vi "SerialNo.vi"(0 "DB serial number IN":string, 2 "Run uninterrupted?":bool) -> (6 "DB serial number OUT":string, 7 "Continue?":bool)   [LabVIEW 2018]
uses:
  globals/QC_RunInformation.vi
panel:
  in  "Comments:":string
  in  "DB Serial No.:":string
  in  "Batch No.:":string
  in  "Device Category:":string(combo)="ATLAS18SS"
  in  "Manufacturer:":string(combo)="Hamamatsu"
  in  "Wafer No.:":string
  in  "Cancel":bool
  in  "OK":bool
  # "ATLAS Serial No."
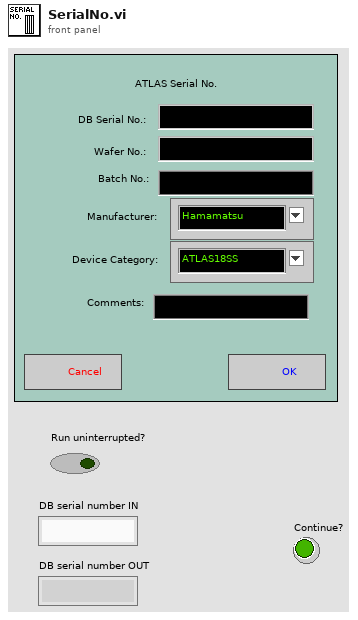
[diagram p1: front panel]
types:
  T1 = cluster{string, string, string, string, string, string, string}
  T2 = cluster{"Institute":string, "Manufacturers":string[], "Devices":string[], "Serialnumbers Lookup DB":string, "Data directory":string, "Backup & screenshot directory":string, "List of known users":string[], "Measurement switch not used":bool, "Measurement Switch":string, "DUT Switch":string, "Rseries IV [MOhm]":string, "Rshunt IV [MOhm]":string, "Rseries CV [MOhm]":string, "DC blocking Cap [µF]":string, "Rseries LCR [MOhm]":string, "Rseries stability [MOhm]":string, "Rshunt stability [MOhm]":string, "Rseries striptest bias [MOhm]":string, "Rseries strip pinhole [MOhm]":string}
  T3 = cluster{"Sensor Serial No.:":string, "Wafer:":string, "Batch:":string, "Manufacturer:":string, "Device Category:":string, "Database Serial No.:":string, "Date Initiated:":string, "Time Initiated:":string, "Test":string, "Probeplan used:":string, "End of Run Status":dbl, "End of Run comment:":string, "User:":string, "Vbias SMU":string, "LCR":string, "Test SMU":string, "Test DMM":string, "Comments":string, "Measurement results":cluster{"IV":string, "CV":string, "Cis":string, "Ris":string, "Stability":string, "PTP":string, "Striptest":string}}
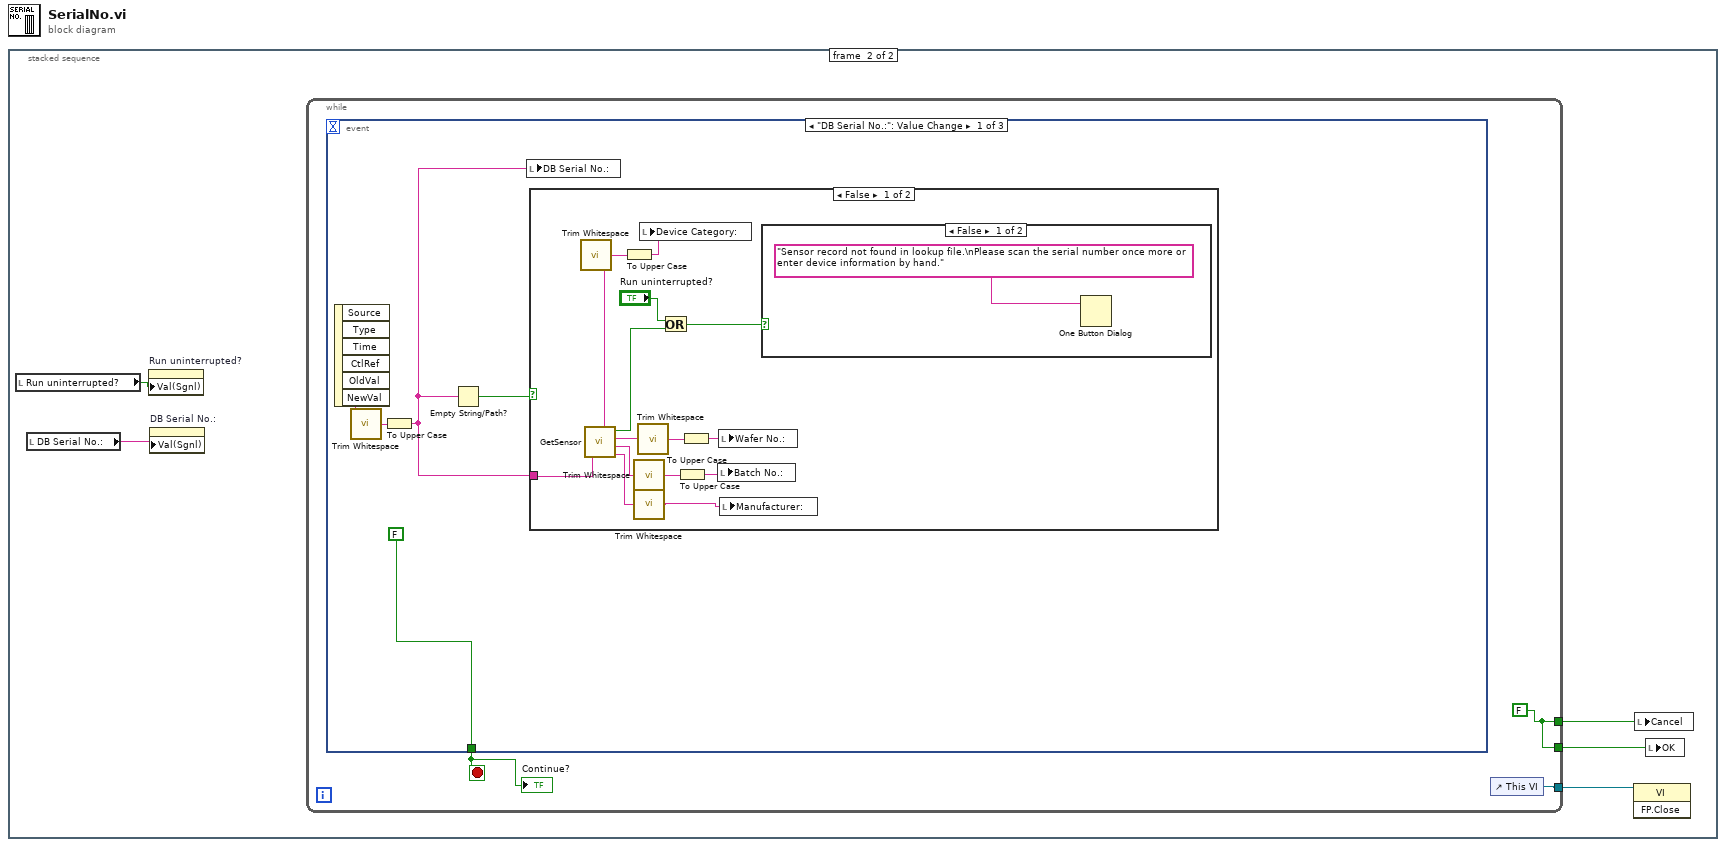
[diagram p0: block diagram]
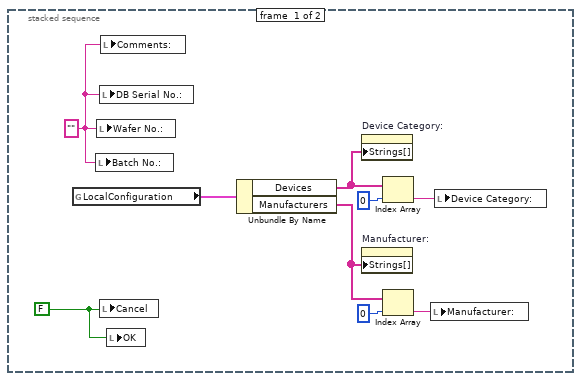
[diagram p2: hidden frame]
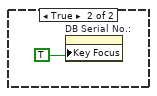
[diagram p4: hidden frame]
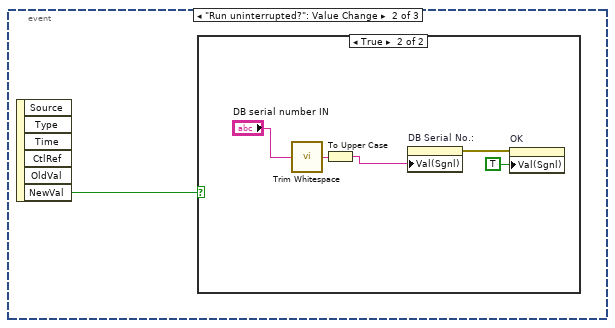
[diagram p5: hidden frame]
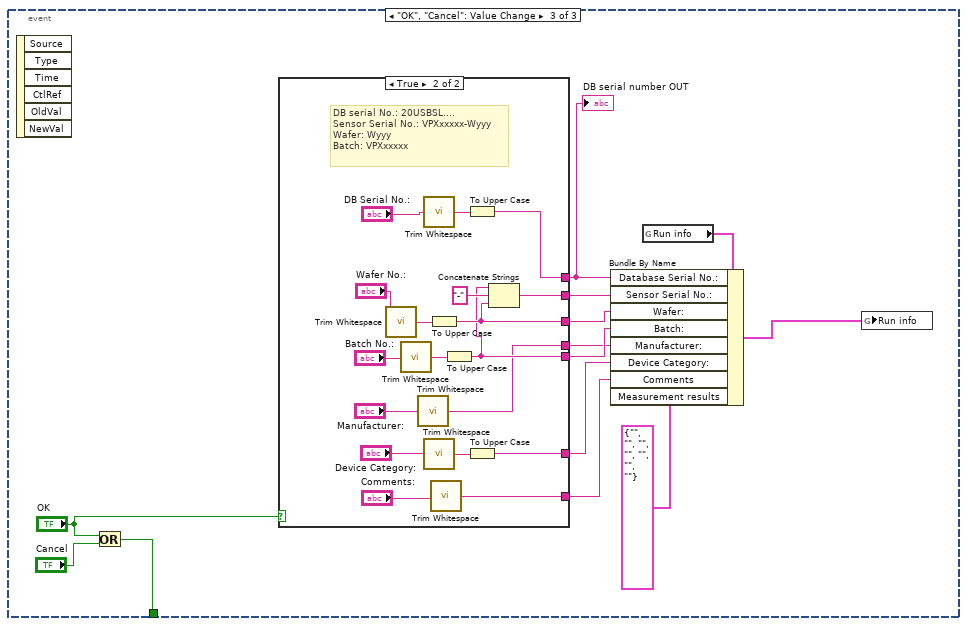
[diagram p7: hidden frame]
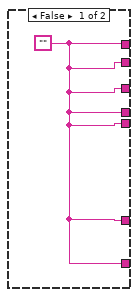
[diagram p8: hidden frame]
diagram:
  n1 = stacked-sequence {
    frame #0 {
      w1 = FALSE
      w2 = ""
      n2 = global read "QC_RunInformation.vi" "LocalConfiguration"() -> (w9:T2)
      n3 = local write "Batch No.:"(w2) -> ()
      n4 = local write "Wafer No.:"(w2) -> ()
      n5 = local write "DB Serial No.:"(w2) -> ()
      n6 = local write "Cancel"(w1) -> ()
      n7 = local write "Comments:"(w2) -> ()
      n8 = local write "OK"(w1) -> ()
      n9 = Unbundle By Name(w9) -> ("Devices"=w4:string[], "Manufacturers"=w3:string[])
      n10 = property on="Device Category:" class="CmbBox"("Strings[]"=w4) -> ()  [unwired: 2 in, 2 out]
      n11 = property on="Manufacturer:" class="CmbBox"("Strings[]"=w3) -> ()  [unwired: 2 in, 2 out]
      n12 = Index Array(array=w4, index=0) -> (element=w5:string)
      n13 = Index Array(array=w3, index=0) -> (element=w6:string)
      n14 = local write "Manufacturer:"(w6) -> ()
      n15 = local write "Device Category:"(w5) -> ()
    }
    frame #1 {
      n16 = local read "Run uninterrupted?"() -> (w14:bool)
      n17 = local read "DB Serial No.:"() -> (w13:string)
      n18 = property on="Run uninterrupted?" class="Bool (strict)"("Val(Sgnl)"=w14) -> ()  [unwired: 2 in, 2 out]
      n19 = property on="DB Serial No.:" class="Str"("Val(Sgnl)"=w13) -> ()  [unwired: 2 in, 2 out]
      n20 = while {
        tunnel: [w17] -> w12
        tunnel: [w16] -> w11
        tunnel: [w16] -> w10
        stop <- w15 stop-if-true
        w16 = FALSE
        n21 = event shown="[0] \"DB Serial No.:\": Value Change" {
          selector: _ -> [_ _ _]
          dyn-events: _ -> [_ _ _]
          timeout: _ -> [_ _ _]
          tunnel: [FALSE ("NewVal") _ w47] -> w15
          event "DB Serial No.:": Value Change {
            n22 = event-data() -> ("NewVal"=w21:string)  [unwired: 1 in, 5 out]
            n23 = call <vilib>:"Trim Whitespace.vi"("string"=w21) -> ("trimmed string"=w22:string)  [unwired: 1 in]
            n24 = To Upper Case(1:w22) -> (0:w20:string)
            n25 = Empty String/Path?(string/path=w20) -> (empty?=w19:bool)
            n26 = local write "DB Serial No.:"(w20) -> ()
            n27 = case shown="False" w19 {
              tunnel: w20 -> [w24 _]
              frame False {
                n28 = call "GetSensor.vi"("DB Serial No. IN"=w24) -> ("Manufacturer"=w33:string, "Batch No."=w31:string, "Wafer No."=w27:string, "Record found?"=w25:bool, "Device Category:"=w36:string)  [unwired: 1 in]
                n29 = call <vilib>:"Trim Whitespace.vi"("string"=w36) -> ("trimmed string"=w35:string)  [unwired: 1 in]
                n30 = To Upper Case(1:w35) -> (0:w37:string)
                n31 = call <vilib>:"Trim Whitespace.vi"("string"=w31) -> ("trimmed string"=w30:string)  [unwired: 1 in]
                n32 = call <vilib>:"Trim Whitespace.vi"("string"=w33) -> ("trimmed string"=w34:string)  [unwired: 1 in]
                n33 = call <vilib>:"Trim Whitespace.vi"("string"=w27) -> ("trimmed string"=w28:string)  [unwired: 1 in]
                n34 = local write "Device Category:"(w37) -> ()
                n35 = Or(x="Run uninterrupted?", y=w25) -> (x .or. y?=w26:bool)
                n36 = To Upper Case(1:w30) -> (0:w32:string)
                n37 = To Upper Case(1:w28) -> (0:w29:string)
                n38 = local write "Batch No.:"(w32) -> ()
                n39 = local write "Wafer No.:"(w29) -> ()
                n40 = local write "Manufacturer:"(w34) -> ()
                n41 = case shown="False" w26 {
                  frame False {
                    n42 = One Button Dialog(message="Sensor record not found in lookup file.\nPlease scan the serial number once more or enter device information by hand.") -> ()  [unwired: 1 in, 1 out]
                  }
                  frame True {
                  }
                }
              }
              frame True {
                n43 = property on="DB Serial No.:" class="Str"("Key Focus"=TRUE) -> ()  [unwired: 2 in, 2 out]
              }
            }
          }
          event "Run uninterrupted?": Value Change {
            n44 = event-data() -> ("NewVal"=w40:bool)  [unwired: 1 in, 5 out]
            n45 = case shown="True" w40 {
              frame False {
              }
              frame True {
                n46 = call <vilib>:"Trim Whitespace.vi"("string"="DB serial number IN") -> ("trimmed string"=w45:string)  [unwired: 1 in]
                n47 = To Upper Case(1:w45) -> (0:w43:string)
                n48 = property on="DB Serial No.:" class="Str"("Val(Sgnl)"=w43) -> (error out=w41:errorcluster)  [unwired: 2 in, 1 out]
                n49 = property on="OK" class="Bool (strict)"(error in=w41, "Val(Sgnl)"=TRUE ("Value (Signaling)")) -> ()  [unwired: 1 in, 2 out]
              }
            }
          }
          event "OK", "Cancel": Value Change {
            n50 = event-data() -> ()  [unwired: 1 in, 6 out]
            n51 = Or(x="OK", y="Cancel") -> (x .or. y?=w47:bool)
            n52 = case shown="True" "OK" {
              tunnel: [w59 w66] -> w50
              tunnel: [w59 w65] -> w57
              tunnel: [w59 w64] -> w56
              tunnel: [w59 w63] -> w55
              tunnel: [w59 w62] -> w54
              tunnel: [w59 w61] -> w53
              tunnel: [w59 w60] -> w52
              frame False {
                w59 = ""
              }
              frame True {
                # "DB serial No.: 20USBSL....\nSensor Serial No.: VPXxxxxx-Wyyy\nWafer: Wyyy\nBatch: VPXxxxxx"
                n53 = call <vilib>:"Trim Whitespace.vi"("string"="Wafer No.:") -> ("trimmed string"=w74:string)  [unwired: 1 in]
                n54 = call <vilib>:"Trim Whitespace.vi"("string"="Batch No.:") -> ("trimmed string"=w72:string)  [unwired: 1 in]
                n55 = call <vilib>:"Trim Whitespace.vi"("string"="Manufacturer:") -> ("trimmed string"=w62:string)  [unwired: 1 in]
                n56 = call <vilib>:"Trim Whitespace.vi"("string"="DB Serial No.:") -> ("trimmed string"=w76:string)  [unwired: 1 in]
                n57 = call <vilib>:"Trim Whitespace.vi"("string"="Device Category:") -> ("trimmed string"=w69:string)  [unwired: 1 in]
                n58 = To Upper Case(1:w74) -> (0:w64:string)
                n59 = call <vilib>:"Trim Whitespace.vi"("string"="Comments:") -> ("trimmed string"=w60:string)  [unwired: 1 in]
                n60 = To Upper Case(1:w72) -> (0:w63:string)
                n61 = To Upper Case(1:w76) -> (0:w66:string)
                n62 = To Upper Case(1:w69) -> (0:w61:string)
                n63 = Concatenate Strings(w63, "-", w64) -> (w65:string)
              }
            }
            "DB serial number OUT" <- w50
            n64 = global read "QC_RunInformation.vi" "Run info"() -> (w51:T3)
            n65 = Bundle By Name(cluster=w51, "Database Serial No.:"=w50, "Sensor Serial No.:"=w57, "Wafer:"=w56, "Batch:"=w55, "Manufacturer:"=w54, "Device Category:"=w53, "Comments"=w52, "Measurement results"=T1 {"", "", "", "", "", "", ""}) -> (w58:T3)
            n66 = global write "QC_RunInformation.vi" "Run info"(w58) -> ()
          }
        }
        "Continue?" <- w15
        n67 = control-ref of="This VI"() -> (w17:refnum<vi>)
      }
      n68 = invoke class="VI" method="FP.Close"(reference=w12) -> ()  [unwired: 2 in, 3 out]
      n69 = local write "Cancel"(w11) -> ()
      n70 = local write "OK"(w10) -> ()
    }
  }
